vi "output.vi"(8 "error in":errorcluster, 10 "output data":T1, 11 "module in":refnum<class "Watchdog runtime.lvclass">) -> (0 "error out":errorcluster, 2 "output allocation":T1, 3 "module out":refnum<class "Watchdog runtime.lvclass">)   [LabVIEW 2013, in "Watchdog runtime.lvclass"]
doc: "Provides an interface for writing data to a module at runtime. While this interface performs no operations, a child should provide an override which may write to any open sessions, references, or interfaces."
uses:
  Watchdog runtime.lvclass
  <vilib>/NI/Tag Bus/table/data table.ctl
  Watchdog runtime.lvclass/Watchdog runtime.ctl
  <vilib>/NI/Tag Bus/table/data table.lvlib
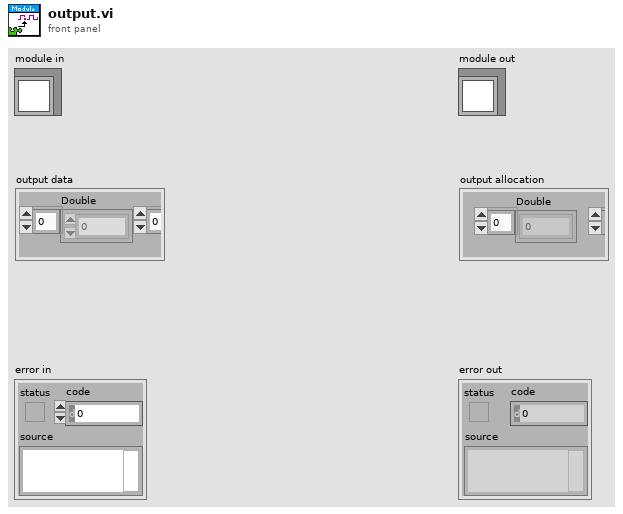
[diagram p1: front panel]
types:
  T1 = typedef "tag bus.lvlib/data table.lvlib/data table.ctl" = cluster{"Double":dbl[], "Single":sgl[], "I64":i64[], "I32":i32[], "I16":i16[], "I8":i8[], "U64":u64[], "U32":u32[], "U16":u16[], "U8":u8[], "Boolean":bool[], "String":string[], "Array of Double":cluster{"DBL Array":dbl[]}[], "Array of Single":cluster{"SGL Array":sgl[]}[], "Array of I64":cluster{"I64 Array":i64[]}[], "Array of I32":cluster{"I32 Array":i32[]}[], "Array of I16":cluster{"I16 Array":i16[]}[], "Array of I8":cluster{"I8 Array":i8[]}[], "Array of U64":cluster{"U64 Array":u64[]}[], "Array of U32":cluster{"U32 Array":u32[]}[], "Array of U16":cluster{"U16 Array":u16[]}[], "Array of U8":cluster{"U8 Array":u8[]}[], "Array of Boolean":cluster{"Boolean Array":bool[]}[], "Array of String":cluster{"String Array":string[]}[]}
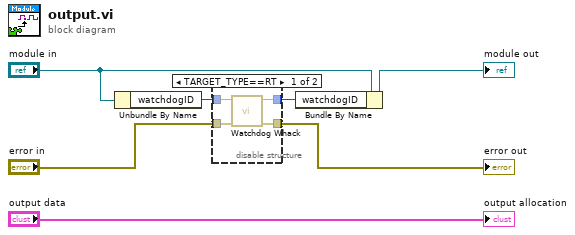
[diagram p0: block diagram]
diagram:
  n1 = Unbundle By Name("module in") -> ("watchdogID"=w7:u32)
  n2 = disable-structure shown="TARGET_TYPE==RT" {
    disable-tunnel: "error in" -> [w11 w13]
    disable-tunnel: [w10 w13] -> w2
    disable-tunnel: w7 -> [w9 w12]
    disable-tunnel: [w8 w12] -> w6
    frame condition #0 {
      n3 = call <vilib>:"Watchdog Whack.vi"("error in (no error)"=w11, "watchdogID in"=w9) -> ("error out"=w10:errorcluster, "watchdogID out"=w8:u32)  [unwired: 3 in, 1 out]
    }
    frame condition #1 (active) {
    }
  }
  "error out" <- w2
  n4 = Bundle By Name(cluster="module in", "watchdogID"=w6) -> (→"module out":refnum<class "Watchdog runtime.lvclass">)
  "output allocation" <- "output data"
